vi "string to tag.vi"(8 "error in":errorcluster, 10 "tag string":string, 11 "tag descriptor in":refnum<class "data bus tag description.lvclass">) -> (0 "error out":errorcluster, 3 "tag descriptor out":refnum<class "data bus tag description.lvclass">)   [LabVIEW 2013, in "data bus tag description.lvclass"]
uses:
  data bus tag description.lvclass
  Data Type.ctl
  data bus tag description.lvclass/data bus tag description.ctl
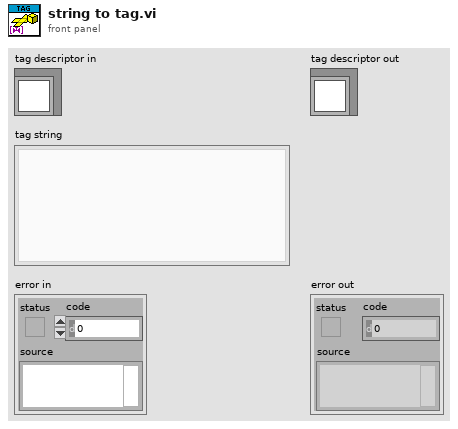
[diagram p1: front panel]
types:
  T1 = cluster{"name":string, "type":string, "default":string, "metadata":string}
  T2 = typedef "data bus tag description.lvclass/Data Type.ctl" = enum16{"Double", "I64", "Boolean", "Array of Double", "Array of I64", "Variant"}
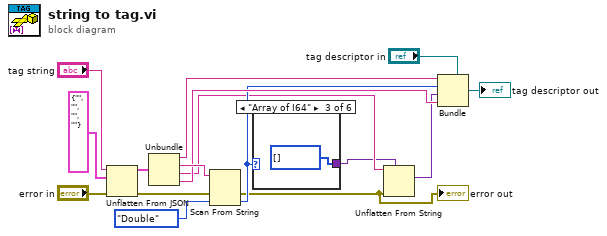
[diagram p0: block diagram]
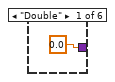
[diagram p2: hidden frame]
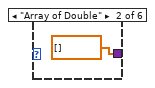
[diagram p3: hidden frame]
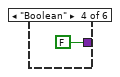
[diagram p4: hidden frame]
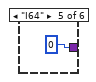
[diagram p5: hidden frame]
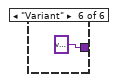
[diagram p6: hidden frame]
diagram:
  n1 = Unflatten From JSON(JSON string="tag string", type and defaults=T1 {"name"="", "type"="", "default"="", "metadata"=""} ("flat tag"), error in (no error)="error in") -> (value=w9:T1, error out=w12:errorcluster)  [unwired: 4 in]
  n2 = Unbundle(w9) -> ("name"=w7:string, "type"=w8:string, "default"=w3:string, "metadata"=w6:string)
  n3 = Scan From String(input string=w8, error in=w12, default 1=Data_Type."Double" ("data type")) -> (error out=w4:errorcluster, output 1=w5:T2)  [unwired: 2 in, 2 out]
  "error out" <- w4
  n4 = case shown="\"Array of I64\"" w5 {
    tunnel: [0.0 dbl[] [] i64[] [] FALSE i64 0 variant ("Variant")] -> w2
    frame "Double" {
    }
    frame "Array of Double" {
    }
    frame "Array of I64" {
    }
    frame "Boolean" {
    }
    frame "I64" {
    }
    frame "Variant" {
    }
  }
  n5 = Unflatten From String(type=w2, binary string=w3, error in (no error)=w4) -> (value=w1:variant)  [unwired: 2 in, 2 out]
  n6 = Bundle(cluster="tag descriptor in", w7, w5, w1, w6) -> (→"tag descriptor out":refnum<class "data bus tag description.lvclass">)
